vi "Find Largest Free Space.vi"(8 "error in (no error)":errorcluster, 9 "border (10)":i16=10, 10 "VI reference":refnum<vi>, 11 "Dialog in":refnum<class "Dialog.lvclass">) -> (0 "error out":errorcluster, 2 "Largest Free Rectangle":T1, 3 "Dialog out":refnum<class "Dialog.lvclass">)   [LabVIEW 2012, in "Dialog.lvlib" / "Dialog.lvclass"]
uses:
  Dialog.lvclass
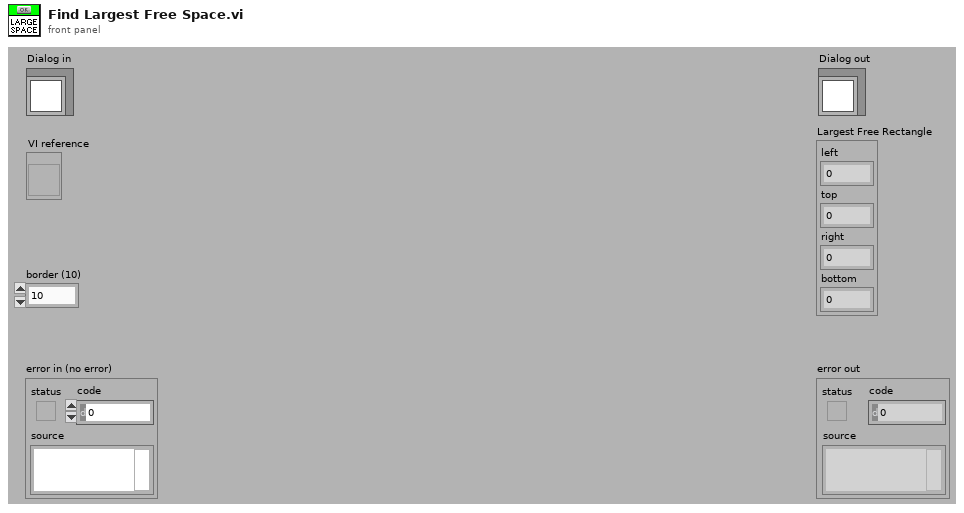
[diagram p1: front panel]
types:
  T1 = cluster{"left":i16, "top":i16, "right":i16, "bottom":i16}
  T2 = cluster{"Area":i32, "Rectangle":cluster{"left":i16, "top":i16, "right":i16, "bottom":i16}}
  T3 = cluster{"Area":i32, "Rectangle":cluster{"left":i16, "top":i16, "right":i16, "bottom":i16}}[]
  T4 = cluster{"Area":i32, "Intersected Rectangle":cluster{"left":i16, "top":i16, "right":i16, "bottom":i16}}
  T5 = cluster{"Area":i32, "Intersected Rectangle":cluster{"left":i16, "top":i16, "right":i16, "bottom":i16}}[]
  T6 = cluster{"left":i16, "top":i16, "right":i16, "bottom":i16}[]
  T7 = cluster{"left":i32, "top":i32, "right":i32, "bottom":i32}
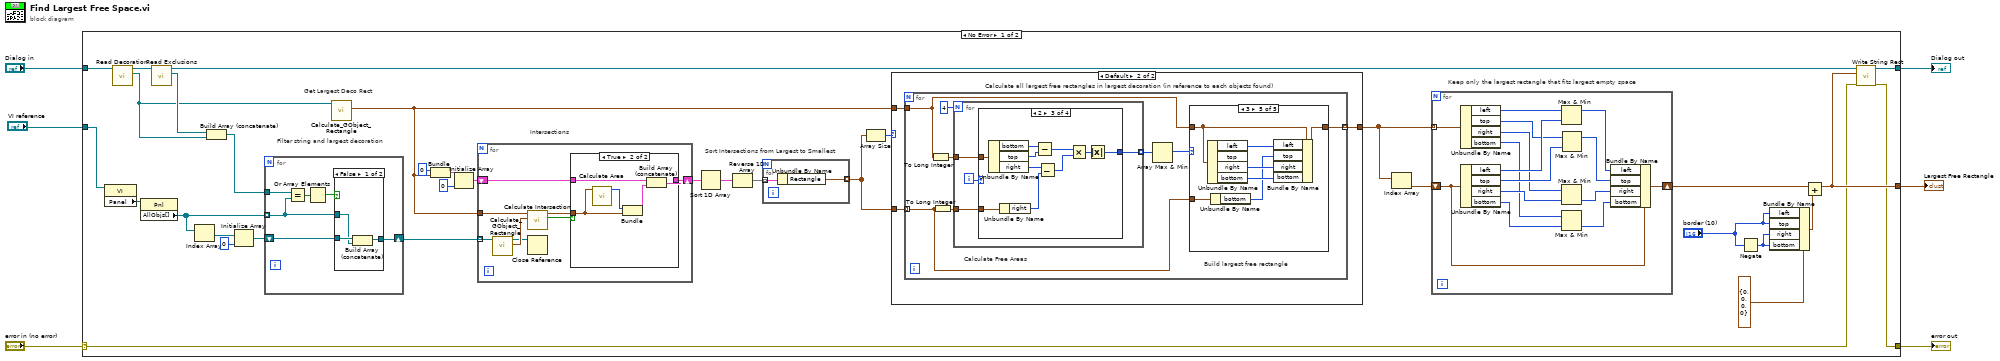
[diagram p0: block diagram]
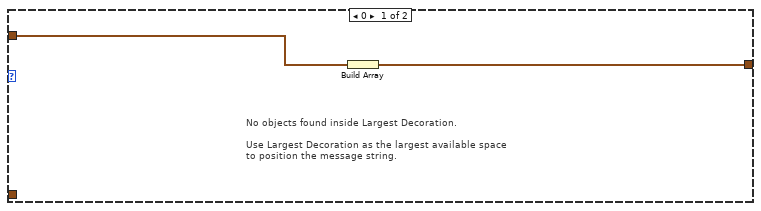
[diagram p2: hidden frame]
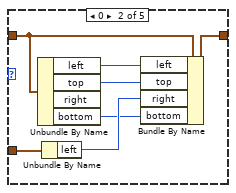
[diagram p4: hidden frame]
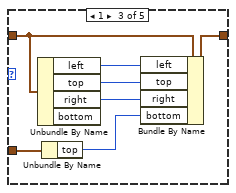
[diagram p5: hidden frame]
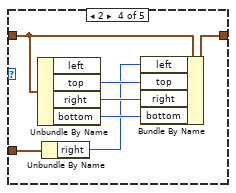
[diagram p6: hidden frame]
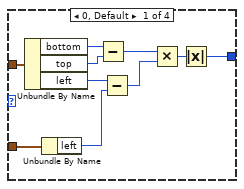
[diagram p7: hidden frame]
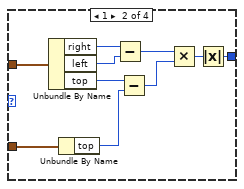
[diagram p8: hidden frame]
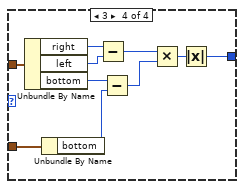
[diagram p9: hidden frame]
diagram:
  n1 = case shown="No Error" "error in (no error)" {
    selector: "error in (no error)" -> [w13 w169]
    tunnel: [w12 w169] -> w5
    tunnel: [w15 w168] -> w3
    tunnel: "Dialog in" -> [w38 w168]
    tunnel: "VI reference" -> [w39 _]
    tunnel: [w14 _] -> w1
    frame No Error {
      # "Keep only the largest rectangle that fits largest empty space"
      # "Sort Intersections from Largest to Smallest"
      # "Intersections"
      # "Get Largest Deco Rect"
      # "Filter string and largest decoration"
      n2 = property class="VI"(reference=w39) -> ("Panel"=w40:refnum<vi>)  [unwired: 1 in, 2 out]
      n3 = call-dynamic "Read Decoration.vi"("Dialog.lvclass in"=w38) -> ("Decoration"=w8:refnum<vi>, "Dialog.lvclass out"=w11:refnum<class "Dialog.lvclass">)  [unwired: 1 in, 8 out]
      n4 = property class="Pnl"(reference=w40) -> ("AllObjs[]"=w35:refnum<vi>[])  [unwired: 1 in, 2 out]
      n5 = call-dynamic "Read Exclusions.vi"("Dialog.lvclass in"=w11) -> ("Exclusions"=w9:refnum<vi>[], "Dialog.lvclass out"=w10:refnum<class "Dialog.lvclass">)  [unwired: 1 in, 8 out]
      n6 = Index Array(array=w35) -> (element=w34:refnum<vi>)  [unwired: 1 in]
      n7 = Build Array (concatenate)(w9, w8) -> (w7:refnum<vi>[])
      n8 = Initialize Array(w34, 0 ("dimension size")) -> (w37:refnum<vi>[])
      n9 = for {
        tunnel: w35 -> [w161] mode=indexing
        shift-right: [w160] -> w31
        shift-left: w37 -> [w162]
        tunnel: w7 -> [w163]
        n10 = Equal?(x=w163, y=w161) -> (x = y?=w159:bool[])
        n11 = Or Array Elements(Boolean array=w159) -> (logical OR=w158:bool)
        n12 = case shown="False" w158 {
          tunnel: w162 -> [w166 w167]
          tunnel: w161 -> [w165 _]
          tunnel: [w164 w167] -> w160
          frame False {
            n13 = Build Array (concatenate)(w166, w165) -> (w164:refnum<vi>[])
          }
          frame True {
          }
        }
      }
      n14 = call "Calculate_GObject_Rectangle.vi"("GObject ref"=w8) -> ("Rectangle"=w27:T1)  [unwired: 1 in, 9 out]
      n15 = Bundle("Area"=0, "Rectangle"=w27) -> (w26:T2)  [unwired: 1 out]
      n16 = Initialize Array(w26, 0 ("dimension size")) -> (w30:T3)
      n17 = for {
        tunnel: w31 -> [w136] mode=indexing
        tunnel: w27 -> [w134]
        shift-right: [w131] -> w25
        shift-left: w30 -> [w132]
        n18 = call "Calculate_GObject_Rectangle.vi"("GObject ref"=w136) -> ("Rectangle"=w135:T1, "GObject ref dup"=w133:refnum<vi>)  [unwired: 1 in, 8 out]
        n19 = call "Calculate Intersection.vi"("Rectangle 2"=w135, "Rectangle"=w134) -> ("Intersection found"=w130:bool, "Intersected Rectangle"=w129:T1)  [unwired: 8 out]
        n20 = Close Reference(reference=w133) -> ()  [unwired: 1 in, 1 out]
        n21 = case shown="True" w130 {
          tunnel: w132 -> [w137 w142]
          tunnel: w129 -> [_ w139]
          tunnel: [w137 w141] -> w131
          frame False {
          }
          frame True {
            n22 = call "Calculate Area.vi"("Rectangle"=w139) -> ("Area"=w140:i32)  [unwired: 10 out]
            n23 = Bundle("Area"=w140, "Intersected Rectangle"=w139) -> (w138:T4)  [unwired: 1 out]
            n24 = Build Array (concatenate)(w142, w138) -> (w141:T5)
          }
        }
      }
      n25 = Sort 1D Array(array=w25) -> (sorted array=w24:T3)
      n26 = Reverse 1D Array(array=w24) -> (reversed array=w23:T3)
      n27 = for {
        tunnel: w23 -> [w128] mode=indexing
        tunnel: [w127] -> w16 mode=indexing
        n28 = Unbundle By Name(w128) -> ("Rectangle"=w127:T1)
      }
      n29 = Array Size(array=w16) -> (size(s)=w17:i32)
      n30 = case shown="Default" w17 {
        tunnel: [w41 w45] -> w33
        tunnel: w27 -> [w42 w44]
        tunnel: w16 -> [_ w43]
        frame 0 {
          # "No objects found inside Largest Decoration.\n\nUse Largest Decoration as the largest available space\nto position the message string."
          n31 = Build Array(w42) -> (w41:T6)
        }
        frame Default {
          # "Calculate all largest free rectangles in largest decoration (in reference to each objects found)"
          n32 = for {
            tunnel: w43 -> [w49] mode=indexing
            tunnel: w44 -> [w47]
            tunnel: [w52] -> w45 mode=indexing
            # "Build largest free rectangle"
            # "Calculate Free Areas"
            n33 = To Long Integer(number=w47) -> (32bit integer=w46:T7)
            n34 = To Long Integer(number=w49) -> (32bit integer=w48:T7)
            n35 = for {
              N: 4 -> [_]
              tunnel: w46 -> [w86]
              tunnel: w48 -> [w85]
              tunnel: [w83] -> w50 mode=indexing
              i -> [w84]
              n36 = case shown="2" w84 {
                tunnel: w86 -> [w96 w98 w116 w126]
                tunnel: w85 -> [w95 w97 w115 w125]
                tunnel: [w87 w99 w107 w117] -> w83
                frame 0, Default {
                  n37 = Unbundle By Name(w96) -> ("bottom"=w93:i32, "top"=w92:i32, "left"=w88:i32)
                  n38 = Unbundle By Name(w95) -> ("left"=w94:i32)
                  n39 = Subtract(x=w93, y=w92) -> (x-y=w91:i32)
                  n40 = Subtract(x=w88, y=w94) -> (x-y=w90:i32)
                  n41 = Multiply(x=w91, y=w90) -> (x*y=w89:i32)
                  n42 = Absolute Value(x=w89) -> (abs(x)=w87:i32)
                }
                frame 1 {
                  n43 = Unbundle By Name(w98) -> ("right"=w105:i32, "left"=w104:i32, "top"=w100:i32)
                  n44 = Unbundle By Name(w97) -> ("top"=w106:i32)
                  n45 = Subtract(x=w105, y=w104) -> (x-y=w103:i32)
                  n46 = Subtract(x=w100, y=w106) -> (x-y=w102:i32)
                  n47 = Multiply(x=w103, y=w102) -> (x*y=w101:i32)
                  n48 = Absolute Value(x=w101) -> (abs(x)=w99:i32)
                }
                frame 2 {
                  n49 = Unbundle By Name(w116) -> ("bottom"=w113:i32, "top"=w112:i32, "right"=w108:i32)
                  n50 = Unbundle By Name(w115) -> ("right"=w114:i32)
                  n51 = Subtract(x=w113, y=w112) -> (x-y=w111:i32)
                  n52 = Subtract(x=w108, y=w114) -> (x-y=w110:i32)
                  n53 = Multiply(x=w111, y=w110) -> (x*y=w109:i32)
                  n54 = Absolute Value(x=w109) -> (abs(x)=w107:i32)
                }
                frame 3 {
                  n55 = Unbundle By Name(w126) -> ("right"=w123:i32, "left"=w122:i32, "bottom"=w118:i32)
                  n56 = Unbundle By Name(w125) -> ("bottom"=w124:i32)
                  n57 = Subtract(x=w123, y=w122) -> (x-y=w121:i32)
                  n58 = Subtract(x=w118, y=w124) -> (x-y=w120:i32)
                  n59 = Multiply(x=w121, y=w120) -> (x*y=w119:i32)
                  n60 = Absolute Value(x=w119) -> (abs(x)=w117:i32)
                }
              }
            }
            n61 = Array Max & Min(array=w50) -> (max index (indices)=w51:i32)  [unwired: 3 out]
            n62 = case shown="3" w51 {
              tunnel: w47 -> [w54 w60 w67 w74 w81]
              tunnel: [w54 w59 w66 w73 w80] -> w52
              tunnel: w49 -> [_ w61 w68 w75 w82]
              frame Default {
              }
              frame 0 {
                n63 = Unbundle By Name(w60) -> ("left"=w58:i16, "top"=w57:i16, "bottom"=w55:i16)  [unwired: 1 out]
                n64 = Unbundle By Name(w61) -> ("left"=w56:i16)
                n65 = Bundle By Name(cluster=w60, "left"=w58, "top"=w57, "right"=w56, "bottom"=w55) -> (w59:T1)
              }
              frame 1 {
                n66 = Unbundle By Name(w67) -> ("left"=w65:i16, "top"=w64:i16, "right"=w63:i16)  [unwired: 1 out]
                n67 = Unbundle By Name(w68) -> ("top"=w62:i16)
                n68 = Bundle By Name(cluster=w67, "left"=w65, "top"=w64, "right"=w63, "bottom"=w62) -> (w66:T1)
              }
              frame 2 {
                n69 = Unbundle By Name(w74) -> ("top"=w72:i16, "right"=w71:i16, "bottom"=w70:i16)  [unwired: 1 out]
                n70 = Unbundle By Name(w75) -> ("right"=w69:i16)
                n71 = Bundle By Name(cluster=w74, "left"=w69, "top"=w72, "right"=w71, "bottom"=w70) -> (w73:T1)
              }
              frame 3 {
                n72 = Unbundle By Name(w81) -> ("left"=w77:i16, "right"=w79:i16, "bottom"=w78:i16)  [unwired: 1 out]
                n73 = Unbundle By Name(w82) -> ("bottom"=w76:i16)
                n74 = Bundle By Name(cluster=w81, "left"=w77, "top"=w76, "right"=w79, "bottom"=w78) -> (w80:T1)
              }
            }
          }
        }
      }
      n75 = Index Array(array=w33) -> (element=w32:T1)  [unwired: 1 in]
      n76 = for {
        tunnel: w33 -> [w157] mode=indexing
        shift-right: [w156] -> w22
        shift-left: w32 -> [w155]
        n77 = Unbundle By Name(w157) -> ("left"=w154:i16, "top"=w151:i16, "right"=w148:i16, "bottom"=w146:i16)
        n78 = Unbundle By Name(w155) -> ("left"=w153:i16, "top"=w150:i16, "right"=w147:i16, "bottom"=w145:i16)
        n79 = Max & Min(x=w154, y=w153) -> (max(x,y)=w152:i16)  [unwired: 1 out]
        n80 = Max & Min(x=w148, y=w147) -> (min(x,y)=w144:i16)  [unwired: 1 out]
        n81 = Max & Min(x=w146, y=w145) -> (min(x,y)=w143:i16)  [unwired: 1 out]
        n82 = Max & Min(x=w151, y=w150) -> (max(x,y)=w149:i16)  [unwired: 1 out]
        n83 = Bundle By Name(cluster=w155, "left"=w152, "top"=w149, "right"=w144, "bottom"=w143) -> (w156:T1)
      }
      n84 = Negate(x="border (10)") -> (-x=w19:i16)
      n85 = Bundle By Name(cluster=T1 {"left"=0, "top"=0, "right"=0, "bottom"=0} ("y"), "left"="border (10)", "top"="border (10)", "right"=w19, "bottom"=w19) -> (w20:T1)
      n86 = Add(x=w22, y=w20) -> (x+y=w14:T1)
      n87 = call-dynamic "Write String Rect.vi"("error in (no error)"=w13, "Object Rect"=w14, "Dialog.lvclass in"=w10) -> ("error out"=w12:errorcluster, "Dialog.lvclass out"=w15:refnum<class "Dialog.lvclass">)  [unwired: 7 out]
    }
    frame Error {
    }
  }
  "error out" <- w5
  "Dialog out" <- w3
  "Largest Free Rectangle" <- w1
